vi "Emballage scan produit a emballer_MEDIC.vi"(0 "nom de ressource VISA":refnum<visa-resource-name>="ASRL3::INSTR", 2 "Tableau des produits":string[][](array[string]), 3 "error in (no error)":errorcluster caption="entrée d'erreur (pas d'erreur)", 4 "Emballage (T)":bool=TRUE) -> (1 "Nom du produit":string, 5 "Output VISA Imprimante":refnum<visa-resource-name>="none", 6 "Test hystérèse (T)":bool, 7 "Arrêter le programme (T)":bool, 8 "Test fuite (T)":bool, 9 "Dec.Droite":string="^LH70,20", 10 "error out":errorcluster caption="sortie d'erreur")   [LabVIEW 2020]
panel:
  in  "Configurer":bool
  in  "Choix imprimante":T1(ring)
  in  "Test hystérèse":bool
  in  "Test fuite":bool
  out "Résultat scanner":string
  in  "liste":bool
  in  "Scanner":bool
  out "Scanner ou liste":string
  in  "Bouton OK":bool
  in  "Annuler?":bool
  in  "Sélectionner un produit:":i32(listbox)
  # "Choix du produit à emballer"
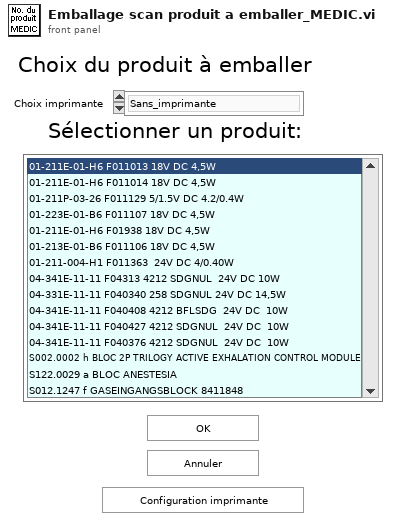
[diagram p1: front panel]
types:
  T1 = enum16{"Sans_imprimante", "Zebra_Medic_emballage2", "Zebra_Medic_2", "Zebra_Medic_1", "Zebra_Flat_emballage"}
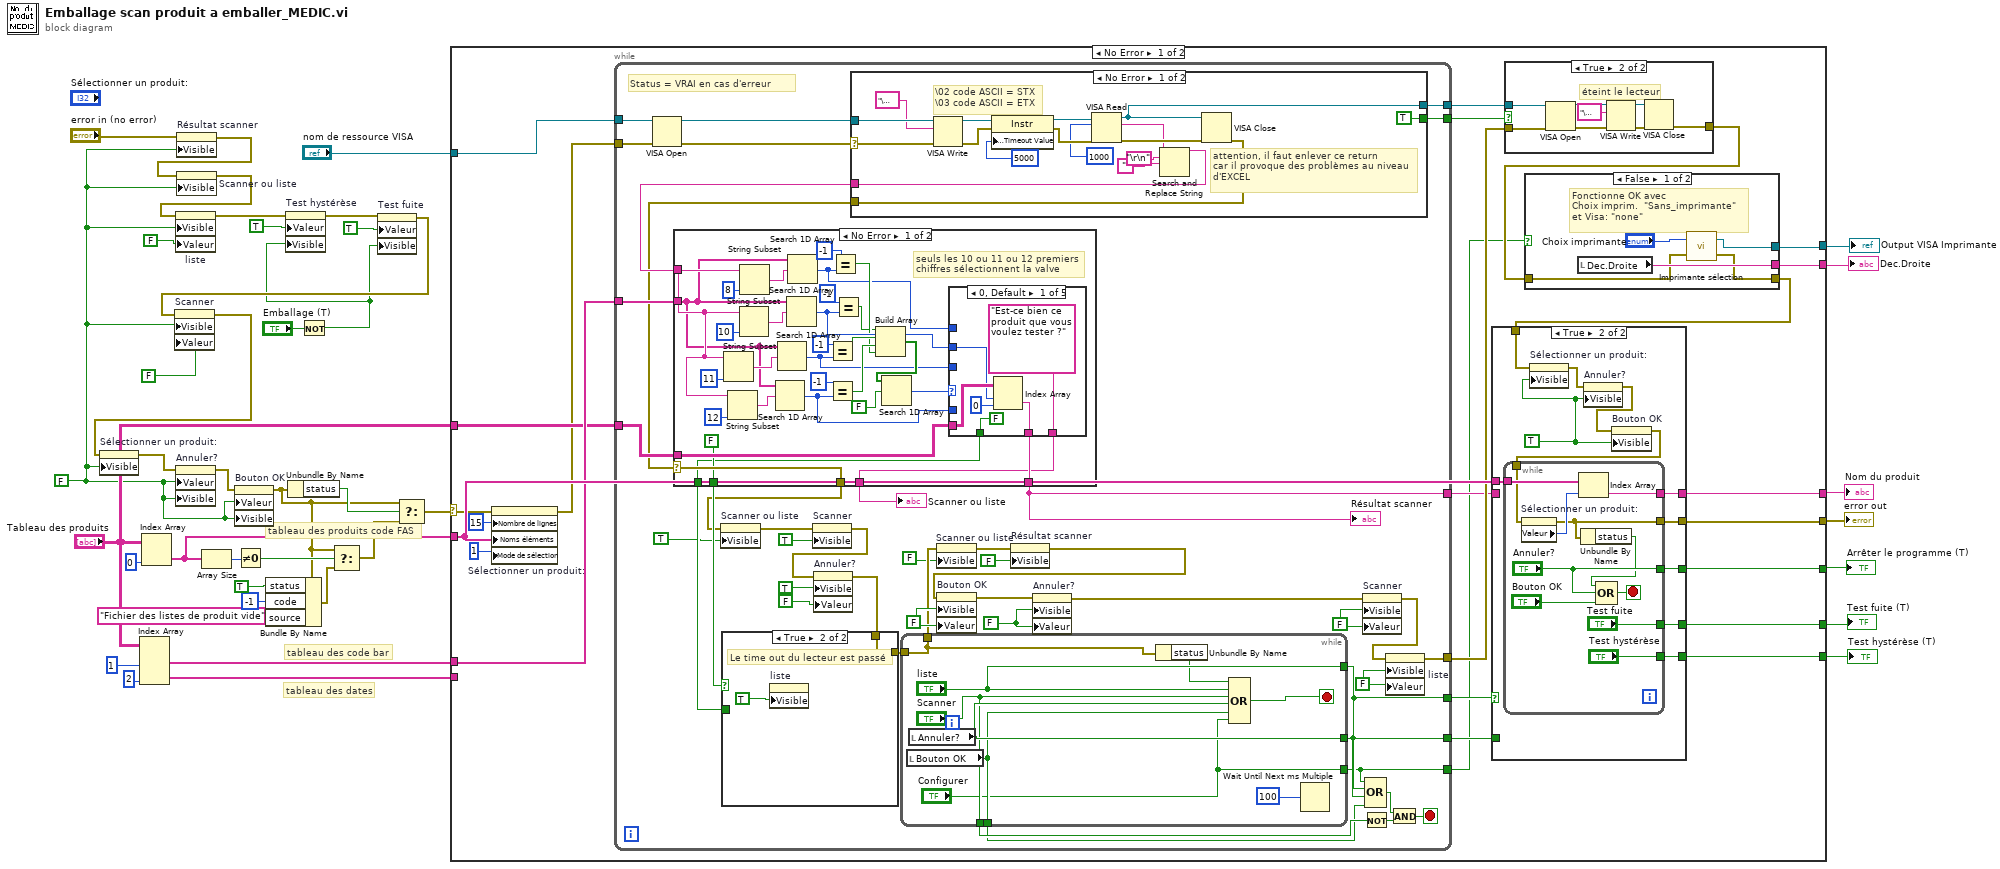
[diagram p0: block diagram]
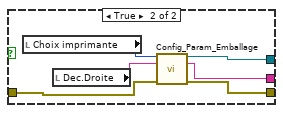
[diagram p3: hidden frame]
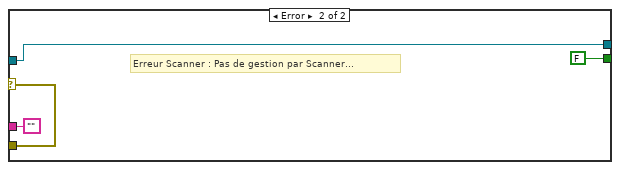
[diagram p4: hidden frame]
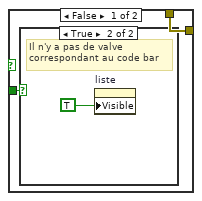
[diagram p5: hidden frame]
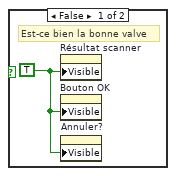
[diagram p6: hidden frame]
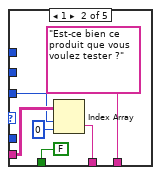
[diagram p7: hidden frame]
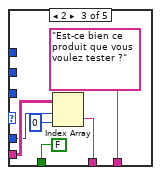
[diagram p8: hidden frame]
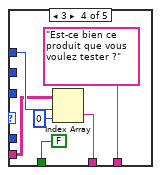
[diagram p9: hidden frame]
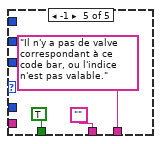
[diagram p10: hidden frame]
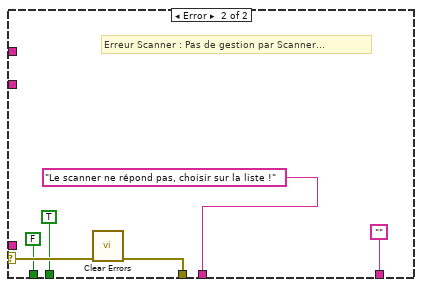
[diagram p11: hidden frame]
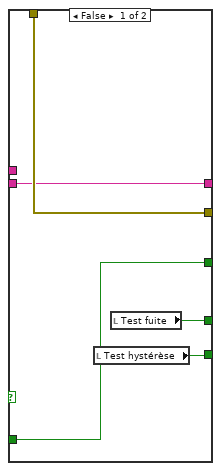
[diagram p12: hidden frame]
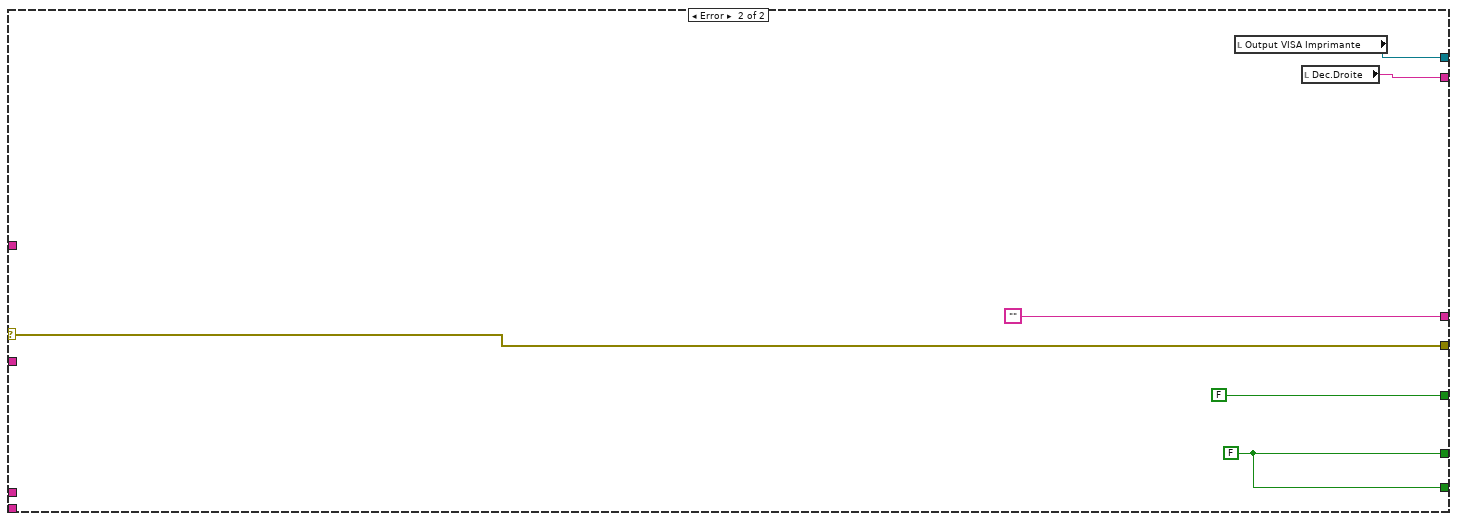
[diagram p13: hidden frame]
diagram:
  w17 = FALSE
  # "tableau des dates"
  # "tableau des produits code FAS"
  # "tableau des code bar"
  n1 = Index Array(array="Tableau des produits", index (col) #1=1, index (col) #2=2) -> (element #1=w22:string[], element #2=w3:string[])  [unwired: 2 in]
  n2 = Index Array(array="Tableau des produits", index (col)=0) -> (element=w25:string[])  [unwired: 1 in]
  n3 = property on="Résultat scanner" class="Str"(error in="error in (no error)", "Visible"=w17) -> (error out=w19:errorcluster)  [unwired: 1 in, 1 out]
  n4 = property on="Scanner ou liste" class="Str"(error in=w19, "Visible"=w17) -> (error out=w18:errorcluster)  [unwired: 1 in, 1 out]
  n5 = property on="liste" class="Bool (strict)"(error in=w18, "Visible"=w17, "Valeur"=FALSE) -> (error out=w11:errorcluster)  [unwired: 1 in, 1 out]
  n6 = Array Size(array=w25) -> (size(s)=w37:i32)
  n7 = Not Equal To 0?(x=w37) -> (x != 0?=w31:bool)
  n8 = Not(x="Emballage (T)") -> (.not. x?=w5:bool)
  n9 = property on="Test hystérèse" class="Bool (strict)"(error in=w11, "Valeur"=TRUE ("Test hystérèse"), "Visible"=w5) -> (error out=w10:errorcluster)  [unwired: 1 in, 1 out]
  n10 = property on="Test fuite" class="Bool (strict)"(error in=w10, "Valeur"=TRUE ("Test fuite"), "Visible"=w5) -> (error out=w9:errorcluster)  [unwired: 1 in, 1 out]
  n11 = property on="Scanner" class="Bool (strict)"(error in=w9, "Visible"=w17, "Valeur"=FALSE) -> (error out=w14:errorcluster)  [unwired: 1 in, 1 out]
  n12 = property on="Sélectionner un produit:" class="LstBox (strict)"(error in=w14, "Visible"=w17) -> (error out=w27:errorcluster)  [unwired: 1 in, 1 out]
  n13 = property on="Annuler?" class="Bool (strict)"(error in=w27, "Valeur"=w17, "Visible"=w17) -> (error out=w40:errorcluster)  [unwired: 1 in, 1 out]
  n14 = property on="Bouton OK" class="Bool (strict)"(error in=w40, "Valeur"=w17, "Visible"=w17) -> (error out=w28:errorcluster)  [unwired: 1 in, 1 out]
  n15 = Bundle By Name(cluster=w28, "status"=TRUE, "code"=-1, "source"="Fichier des listes de produit vide") -> (w30:errorcluster)
  n16 = Unbundle By Name(w28) -> ("status"=w33:bool)
  n17 = Select(t=w28, s=w31, f=w30) -> (s? t:f=w29:errorcluster)
  n18 = Select(t=w28, s=w33, f=w29) -> (s? t:f=w32:errorcluster)
  n19 = case shown="No Error" w32 {
    selector: w32 -> [w61 w262]
    tunnel: [w63 w262] -> w41
    tunnel: w25 -> [w62 _]
    tunnel: [w60 FALSE] -> w38
    tunnel: [w59 ""] -> w39
    tunnel: "nom de ressource VISA" -> [w56 _]
    tunnel: w22 -> [w55 _]
    tunnel: "Tableau des produits" -> [w54 _]
    tunnel: [w49 w259] -> w8
    tunnel: [w48 w259] -> w7
    tunnel: w3 -> [_ _]
    tunnel: [w44 w258] -> w2
    tunnel: [w43 w257] -> w1
    frame No Error {
      n20 = property on="Sélectionner un produit:" class="LstBox (strict)"(error in=w61, "Nombre de lignes"=15, "Noms éléments"=w62, "Mode de sélection"=1) -> (error out=w53:errorcluster)  [unwired: 1 in, 1 out]
      n21 = while {
        tunnel: w56 -> [w128]
        tunnel: w53 -> [w127]
        tunnel: [w110] -> w57
        tunnel: [w104] -> w58
        tunnel: [w91] -> w51
        tunnel: w55 -> [w126]
        tunnel: w54 -> [w124]
        tunnel: [w108] -> w52
        tunnel: [w109] -> w50
        tunnel: [w89] -> w45
        tunnel: [w86] -> w42
        stop <- w114 stop-if-true
        w100 = FALSE
        w101 = FALSE
        w102 = FALSE
        w103 = FALSE
        # "Status = VRAI en cas d'erreur"
        n22 = VISA Open(error in (no error)=w127, VISA resource name=w128) -> (VISA resource name=w129:refnum<visa-resource-name>, error out=w87:errorcluster)  [unwired: 3 in]
        n23 = case shown="No Error" w87 {
          selector: w87 -> [w131 w149]
          tunnel: w129 -> [w146 w150]
          tunnel: [w134 "" ("result string")] -> w125
          tunnel: [w133 w150] -> w91
          tunnel: [w132 w149] -> w88
          tunnel: [TRUE FALSE] -> w86
          frame No Error {
            # "attention, il faut enlever ce return\ncar il provoque des problèmes au niveau\nd'EXCEL"
            # "\\02 code ASCII = STX\n\\03 code ASCII = ETX"
            n24 = VISA Write(VISA resource name=w146, write buffer="\u0002", error in (no error)=w131) -> (VISA resource name out=w144:refnum<visa-resource-name>, error out=w145:errorcluster)  [unwired: 1 out]
            n25 = property class="Instr"(reference=w144, error in=w145, "General Settings:Timeout Value"=u32 5000 ("Tmo Value")) -> (reference out=w142:refnum<visa-resource-name>, error out=w143:errorcluster)
            n26 = VISA Read(VISA resource name=w142, byte count=u32 1000 ("byte count (0)"), error in (no error)=w143) -> (VISA resource name out=w133:refnum<visa-resource-name>, read buffer=w138:string, error out=w139:errorcluster)  [unwired: 1 out]
            n27 = Search and Replace String(input string=w138, search string="\r\n", replace string="") -> (result string=w134:string)  [unwired: 5 in, 3 out]
            n28 = VISA Close(VISA resource name=w133, error in (no error)=w139) -> (error out=w132:errorcluster)
          }
          frame Error {
            # "Erreur Scanner : Pas de gestion par Scanner..."
          }
        }
        n29 = case shown="No Error" w88 {
          selector: w88 -> [w196 w229]
          tunnel: [w196 w225] -> w120
          tunnel: [w192 "Le scanner ne répond pas, choisir sur la liste !"] -> w122
          tunnel: w126 -> [w170 _]
          tunnel: w125 -> [w171 _]
          tunnel: w124 -> [w195 _]
          tunnel: [w174 FALSE] -> w123
          tunnel: [FALSE TRUE] -> w121
          tunnel: [w193 ""] -> w109
          frame No Error {
            # "seuls les 10 ou 11 ou 12 premiers \nchiffres sélectionnent la valve"
            n30 = String Subset(string=w171, length (rest)=11 ("longueur (reste)")) -> (substring=w187:string)  [unwired: 1 in]
            n31 = String Subset(string=w171, length (rest)=12 ("longueur (reste)")) -> (substring=w185:string)  [unwired: 1 in]
            n32 = String Subset(string=w171, length (rest)=10 ("longueur (reste)")) -> (substring=w188:string)  [unwired: 1 in]
            n33 = String Subset(string=w171, length (rest)=8 ("longueur (reste)")) -> (substring=w172:string)  [unwired: 1 in]
            n34 = Search 1D Array(1D array=w170, element=w185) -> (index of element=w175:i32)  [unwired: 1 in]
            n35 = Search 1D Array(1D array=w170, element=w187) -> (index of element=w176:i32)  [unwired: 1 in]
            n36 = Search 1D Array(1D array=w170, element=w188) -> (index of element=w177:i32)  [unwired: 1 in]
            n37 = Search 1D Array(1D array=w170, element=w172) -> (index of element=w167:i32)  [unwired: 1 in]
            n38 = Equal?(x=-1, y=w176) -> (x = y?=w182:bool)
            n39 = Equal?(x=-1, y=w175) -> (x = y?=w181:bool)
            n40 = Equal?(x=-1, y=w167) -> (x = y?=w168:bool)
            n41 = Equal?(x=-1, y=w177) -> (x = y?=w166:bool)
            n42 = Build Array(w166, w182, w181, w168) -> (w180:bool[])
            n43 = Search 1D Array(1D array=w180, element=FALSE ("élément")) -> (index of element=w178:i32)  [unwired: 1 in]
            n44 = case shown="0, Default" w178 {
              tunnel: w195 -> [w201 w207 w213 w215 _]
              tunnel: ["Est-ce bien ce produit que vous voulez tester ?" "Est-ce bien ce produit que vous voulez tester ?" "Est-ce bien ce produit que vous voulez tester ?" "Est-ce bien ce produit que vous voulez tester ?" "Il n'y a pas de valve correspondant à ce code bar, ou l'indice n'est pas valable."] -> w192
              tunnel: [w200 w206 w212 w218 ""] -> w193
              tunnel: w177 -> [w198 _ _ _ _]
              tunnel: w176 -> [_ w204 _ _ _]
              tunnel: w175 -> [_ _ w210 _ _]
              tunnel: [FALSE FALSE FALSE FALSE TRUE] -> w174
              tunnel: w167 -> [_ _ _ w216 _]
              frame 0, Default {
                n45 = Index Array(array=w201, index (row)=w198, index (col)=0) -> (element=w200:string)
              }
              frame 1 {
                n46 = Index Array(array=w207, index (row)=w204, index (col)=0) -> (element=w206:string)
              }
              frame 2 {
                n47 = Index Array(array=w213, index (row)=w210, index (col)=0) -> (element=w212:string)
              }
              frame 3 {
                n48 = Index Array(array=w215, index (row)=w216, index (col)=0) -> (element=w218:string)
              }
              frame -1 {
              }
            }
          }
          frame Error {
            # "Erreur Scanner : Pas de gestion par Scanner..."
            n49 = call <vilib>:"Clear Errors.vi"("error in (no error)"=w229) -> ("error out"=w225:errorcluster)  [unwired: 5 in, 1 out]
          }
        }
        "Scanner ou liste" <- w122
        "Résultat scanner" <- w109
        n50 = property on="Scanner ou liste" class="Str"(error in=w120, "Visible"=TRUE) -> (error out=w118:errorcluster)  [unwired: 1 in, 1 out]
        n51 = property on="Scanner" class="Bool (strict)"(error in=w118, "Visible"=TRUE) -> (error out=w93:errorcluster)  [unwired: 1 in, 1 out]
        n52 = property on="Annuler?" class="Bool (strict)"(error in=w93, "Visible"=TRUE, "Valeur"=FALSE) -> (error out=w92:errorcluster)  [unwired: 1 in, 1 out]
        n53 = case shown="True" w121 {
          tunnel: w92 -> [w161 w165]
          tunnel: [w161 w165] -> w116
          tunnel: w123 -> [w160 _]
          frame False {
            n54 = case shown="True" w160 {
              frame False {
                w162 = TRUE
                # "Est-ce bien la bonne valve"
                n55 = property on="Résultat scanner" class="Str"("Visible"=w162) -> ()  [unwired: 2 in, 2 out]
                n56 = property on="Bouton OK" class="Bool (strict)"("Visible"=w162) -> ()  [unwired: 2 in, 2 out]
                n57 = property on="Annuler?" class="Bool (strict)"("Visible"=w162) -> ()  [unwired: 2 in, 2 out]
              }
              frame True {
                # "Il n'y a pas de valve\ncorrespondant au code bar"
                n58 = property on="liste" class="Bool (strict)"("Visible"=TRUE) -> ()  [unwired: 2 in, 2 out]
              }
            }
          }
          frame True {
            # "Le time out du lecteur est passé"
            n59 = property on="liste" class="Bool (strict)"("Visible"=TRUE) -> ()  [unwired: 2 in, 2 out]
          }
        }
        n60 = while {
          tunnel: [w157] -> w108
          tunnel: ["liste"] -> w110
          tunnel: w116 -> [w152]
          tunnel: [w152] -> w99
          tunnel: [w155] -> w111
          tunnel: ["Scanner"] -> w112
          tunnel: ["Configurer"] -> w89
          stop <- w159 stop-if-true
          n61 = local read "Bouton OK"() -> (w155:bool)
          n62 = local read "Annuler?"() -> (w157:bool)
          n63 = Unbundle By Name(w152) -> ("status"=w153:bool)
          n64 = Compound Arithmetic op=OR(w153, "liste", "Scanner", w157, w155, "Configurer") -> (w159:bool)
          n65 = Wait Until Next ms Multiple(millisecond multiple=100) -> ()  [unwired: 1 out]
        }
        n66 = property on="Scanner ou liste" class="Str"(error in=w99, "Visible"=FALSE) -> (error out=w98:errorcluster)  [unwired: 1 in, 1 out]
        n67 = property on="Résultat scanner" class="Str"(error in=w98, "Visible"=FALSE) -> (error out=w97:errorcluster)  [unwired: 1 in, 1 out]
        n68 = property on="Bouton OK" class="Bool (strict)"(error in=w97, "Visible"=w100, "Valeur"=w100) -> (error out=w107:errorcluster)  [unwired: 1 in, 1 out]
        n69 = property on="Annuler?" class="Bool (strict)"(error in=w107, "Visible"=w101, "Valeur"=w101) -> (error out=w106:errorcluster)  [unwired: 1 in, 1 out]
        n70 = Not(x=w112) -> (.not. x?=w113:bool)
        n71 = property on="Scanner" class="Bool (strict)"(error in=w106, "Visible"=w102, "Valeur"=w102) -> (error out=w105:errorcluster)  [unwired: 1 in, 1 out]
        n72 = Compound Arithmetic op=OR(w89, w110, w108, w111) -> (w115:bool)
        n73 = property on="liste" class="Bool (strict)"(error in=w105, "Visible"=w103, "Valeur"=w103) -> (error out=w104:errorcluster)  [unwired: 1 in, 1 out]
        n74 = And(x=w115, y=w113) -> (x .and. y?=w114:bool)
      }
      n75 = case shown="True" w42 {
        tunnel: w58 -> [w66 w69]
        tunnel: w51 -> [_ w68]
        tunnel: [w66 w67] -> w47
        frame False {
        }
        frame True {
          # "éteint le lecteur"
          n76 = VISA Open(error in (no error)=w69, VISA resource name=w68) -> (VISA resource name=w71:refnum<visa-resource-name>, error out=w73:errorcluster)  [unwired: 3 in]
          n77 = VISA Write(VISA resource name=w71, write buffer="\u0003", error in (no error)=w73) -> (VISA resource name out=w70:refnum<visa-resource-name>, error out=w72:errorcluster)  [unwired: 1 out]
          n78 = VISA Close(VISA resource name=w70, error in (no error)=w72) -> (error out=w67:errorcluster)
        }
      }
      n79 = case shown="False" w45 {
        tunnel: [w75 w84] -> w43
        tunnel: [w79 w83] -> w44
        tunnel: w47 -> [w77 w82]
        tunnel: [w76 w81] -> w46
        frame False {
          # "Fonctionne OK avec \nChoix imprim.  \"Sans_imprimante\"\net Visa: \"none\""
          n80 = local read "Dec.Droite"() -> (w79:string)
          n81 = call "Imprimante sélection.vi"("entrée d'erreur"=w77, "Choix imprimante"="Choix imprimante") -> ("sortie d'erreur"=w76:errorcluster, "Output ressource VISA"=w75:refnum<visa-resource-name>)
        }
        frame True {
          n82 = local read "Choix imprimante"() -> (w80:T1)
          n83 = local read "Dec.Droite"() -> (w85:string)
          n84 = call "Config_Param_Emballage.vi"("Choix imprimante"=w80, "Dec.Droite"=w85, "error in (no error)"=w82) -> ("Output VISA Imprimante"=w84:refnum<visa-resource-name>, "New_Dec.Droite"=w83:string, "error out"=w81:errorcluster)  [unwired: 10 in]
        }
      }
      n85 = case shown="True" w57 {
        tunnel: [w233 w245] -> w63
        tunnel: w62 -> [_ w244]
        tunnel: [w234 w243] -> w60
        tunnel: [w232 w242] -> w59
        tunnel: w52 -> [w234 _]
        tunnel: w46 -> [w233 w240]
        tunnel: w50 -> [w232 _]
        tunnel: [w231 w236] -> w49
        tunnel: [w230 w235] -> w48
        frame False {
          n86 = local read "Test hystérèse"() -> (w230:bool)
          n87 = local read "Test fuite"() -> (w231:bool)
        }
        frame True {
          w241 = TRUE
          n88 = property on="Sélectionner un produit:" class="LstBox (strict)"(error in=w240, "Visible"=w241) -> (error out=w239:errorcluster)  [unwired: 1 in, 1 out]
          n89 = property on="Annuler?" class="Bool (strict)"(error in=w239, "Visible"=w241) -> (error out=w237:errorcluster)  [unwired: 1 in, 1 out]
          n90 = property on="Bouton OK" class="Bool (strict)"(error in=w237, "Visible"=w241) -> (error out=w238:errorcluster)  [unwired: 1 in, 1 out]
          n91 = while {
            tunnel: ["Annuler?"] -> w243
            tunnel: [w249] -> w245
            tunnel: w244 -> [w255]
            tunnel: w238 -> [w254]
            tunnel: [w253] -> w242
            tunnel: ["Test fuite"] -> w236
            tunnel: ["Test hystérèse"] -> w235
            stop <- w252 stop-if-true
            n92 = property on="Sélectionner un produit:" class="LstBox (strict)"(error in=w254) -> (error out=w249:errorcluster, "Valeur"=w256:i32)  [unwired: 1 in, 1 out]
            n93 = Index Array(array=w255, index=w256) -> (element=w253:string)
            n94 = Unbundle By Name(w249) -> ("status"=w248:bool)
            n95 = Compound Arithmetic op=OR(w248, "Annuler?", "Bouton OK") -> (w252:bool)
          }
        }
      }
    }
    frame Error {
      w259 = FALSE ("Test fuite")
      n96 = local read "Output VISA Imprimante"() -> (w257:refnum<visa-resource-name>)
      n97 = local read "Dec.Droite"() -> (w258:string)
    }
  }
  "error out" <- w41
  "Arrêter le programme (T)" <- w38
  "Nom du produit" <- w39
  "Test fuite (T)" <- w8
  "Test hystérèse (T)" <- w7
  "Dec.Droite" <- w2
  "Output VISA Imprimante" <- w1
